vi "Get Target Data.vi"() -> (0 "y angle":u16, 1 "x angle":u16, 3 "values":dbl[](array[numeric]))   [LabVIEW 2012]
panel:
  out "Val":bool
  in  "Color":string(combo)="YELLOW"
  in  "variables":string[](array[string])=["HORIZ_ANGLE", "VERT_ANGLE", "DISTANCE"]
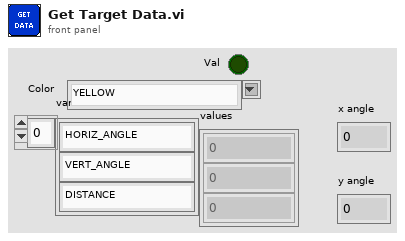
[diagram p1: front panel]
types:
  T1 = typedef "WPI_ServoDeviceRef.ctl" = cluster{"DeviceStatus":errorcluster, "Digital Module":T2, "PWM Channel":T3, "DeadBand":T4}
  T2 = typedef "FPGA_TypedefDigitalModule.ctl" = enum16{"Digital Module 1", "Digital Module 2"}
  T3 = typedef "FPGA_DIOPWMChannel.ctl" = enum8{"PWM 1", "PWM 2", "PWM 3", "PWM 4", "PWM 5", "PWM 6", "PWM 7", "PWM 8", "PWM 9", "PWM 10", "Invalid"}
  T4 = typedef "WPI_PWMDeadband.ctl" = cluster{"Name":string, "maxPositivePwm":i32, "minPositivePwm":i32, "centerPwm":i32, "maxNegativePwm":i32, "minNegativePwm":i32, "angularRange":u16}
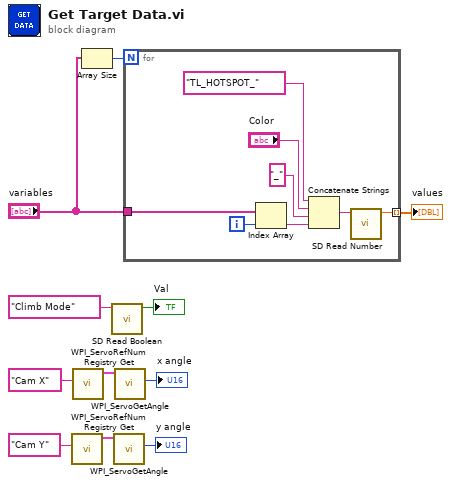
[diagram p0: block diagram]
diagram:
  n1 = call <vilib>:"WPI_ServoRefNum Registry Get.vi"("refnum name"="Cam Y") -> ("ServoDeviceRef"=w3:T1)  [unwired: 9 in, 1 out]
  n2 = call <vilib>:"WPI_ServoRefNum Registry Get.vi"("refnum name"="Cam X") -> ("ServoDeviceRef"=w6:T1)  [unwired: 9 in, 1 out]
  n3 = Array Size(array="variables") -> (size(s)=w11:i32)
  n4 = call <vilib>:"SD Read Boolean.vi"("Name"="Climb Mode") -> ("Boolean"=→"Val":bool)  [unwired: 8 in, 2 out]
  n5 = call <vilib>:"WPI_ServoGetAngle.vi"("ServoDeviceRef"=w3) -> ("Angle"=→"y angle":u16)  [unwired: 7 in, 2 out]
  n6 = call <vilib>:"WPI_ServoGetAngle.vi"("ServoDeviceRef"=w6) -> ("Angle"=→"x angle":u16)  [unwired: 7 in, 2 out]
  n7 = for {
    N: w11 -> [_]
    tunnel: "variables" -> [w17]
    tunnel: [w15] -> w9 mode=indexing
    i -> [w16]
    n8 = Index Array(array=w17, index=w16) -> (element=w14:string)
    n9 = Concatenate Strings("TL_HOTSPOT_" ("Name"), "Color", "_" ("string"), w14) -> (w18:string)
    n10 = call <vilib>:"SD Read Number.vi"("Name"=w18) -> ("Numeric"=w15:dbl)  [unwired: 8 in, 2 out]
  }
  "values" <- w9
